vi "Mail test file V1.vi"(8 "mail file":bool, 9 "result":bool, 10 "status":string, 11 "panel id":string) -> (0 "network file save error":errorcluster, 3 "file save path":string)   [LabVIEW 2013]
uses:
  program files/Global 1.vi
panel:
  in  "mail to":string
  in  "mail from":string
  in  "mail server":string
  out "C drive root path":string
  out "network file dir path":path
  out "network dir":string
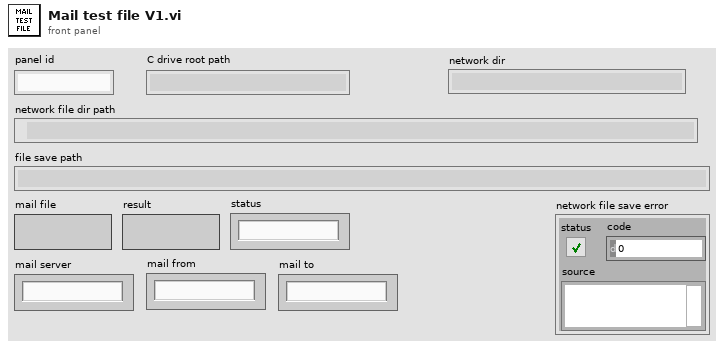
[diagram p1: front panel]
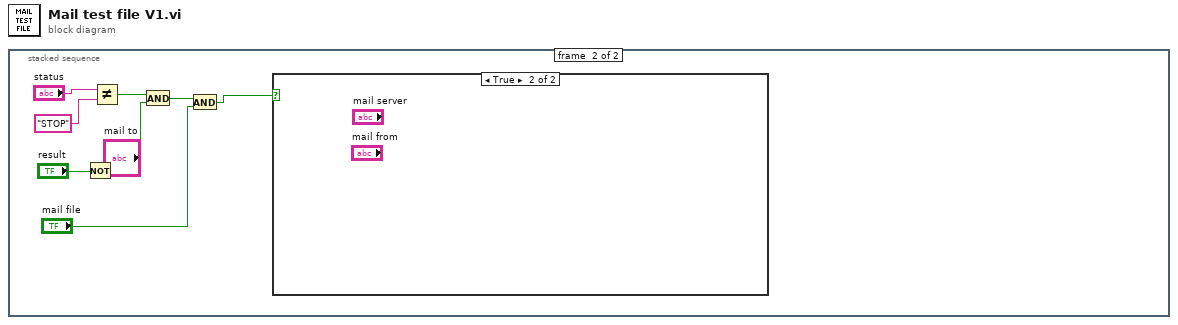
[diagram p0: block diagram]
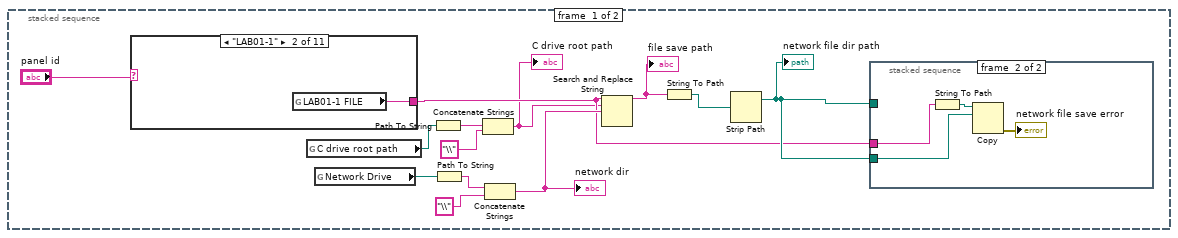
[diagram p2: hidden frame]
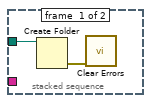
[diagram p3: hidden frame]
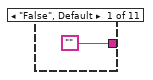
[diagram p4: hidden frame]
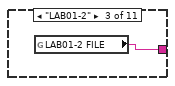
[diagram p5: hidden frame]
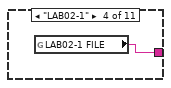
[diagram p6: hidden frame]
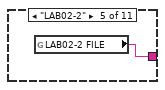
[diagram p7: hidden frame]
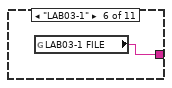
[diagram p8: hidden frame]
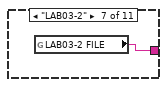
[diagram p9: hidden frame]
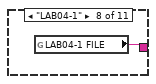
[diagram p10: hidden frame]
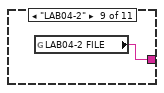
[diagram p11: hidden frame]
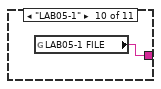
[diagram p12: hidden frame]
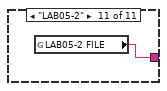
[diagram p13: hidden frame]
diagram:
  n1 = stacked-sequence {
    frame #0 {
      n2 = case shown="\"LAB01-1\"" "panel id" {
        tunnel: ["" w21 w22 w23 w24 w25 w26 w27 w28 w29 w30] -> w5
        frame "False", Default {
        }
        frame "LAB01-1" {
          n3 = global read "Global 1.vi" "LAB01-1 FILE"() -> (w21:string)
        }
        frame "LAB01-2" {
          n4 = global read "Global 1.vi" "LAB01-2 FILE"() -> (w22:string)
        }
        frame "LAB02-1" {
          n5 = global read "Global 1.vi" "LAB02-1 FILE"() -> (w23:string)
        }
        frame "LAB02-2" {
          n6 = global read "Global 1.vi" "LAB02-2 FILE"() -> (w24:string)
        }
        frame "LAB03-1" {
          n7 = global read "Global 1.vi" "LAB03-1 FILE"() -> (w25:string)
        }
        frame "LAB03-2" {
          n8 = global read "Global 1.vi" "LAB03-2 FILE"() -> (w26:string)
        }
        frame "LAB04-1" {
          n9 = global read "Global 1.vi" "LAB04-1 FILE"() -> (w27:string)
        }
        frame "LAB04-2" {
          n10 = global read "Global 1.vi" "LAB04-2 FILE"() -> (w28:string)
        }
        frame "LAB05-1" {
          n11 = global read "Global 1.vi" "LAB05-1 FILE"() -> (w29:string)
        }
        frame "LAB05-2" {
          n12 = global read "Global 1.vi" "LAB05-2 FILE"() -> (w30:string)
        }
      }
      n13 = global read "Global 1.vi" "C drive root path"() -> (w2:path)
      n14 = global read "Global 1.vi" "Network Drive"() -> (w12:path)
      n15 = Path To String(path=w2) -> (string=w3:string)
      n16 = Path To String(path=w12) -> (string=w11:string)
      n17 = Concatenate Strings(w3, "\\") -> (w1:string)
      "C drive root path" <- w1
      n18 = Concatenate Strings(w11, "\\") -> (w9:string)
      "network dir" <- w9
      n19 = Search and Replace String(input string=w5, search string=w1, replace string=w9) -> (result string=w8:string)  [unwired: 5 in, 3 out]
      "file save path" <- w8
      n20 = String To Path(string=w8) -> (path=w7:path)
      n21 = Strip Path(path=w7) -> (stripped path=w6:path)  [unwired: 1 out]
      "network file dir path" <- w6
      n22 = stacked-sequence {
        tunnel: w6 -> [w15 _]
        tunnel: w5 -> [_ w17]
        tunnel: w6 -> [_ w16]
        frame #0 {
          n23 = Create Folder(path (use dialog)=w15) -> (error out=w14:errorcluster)  [unwired: 2 in, 2 out]
          n24 = call <vilib>:"Clear Errors.vi"("error in (no error)"=w14) -> ()  [unwired: 6 in, 1 out]
        }
        frame #1 {
          n25 = String To Path(string=w17) -> (path=w18:path)
          n26 = Copy(10:w16, 11:w18) -> (0:→"network file save error":errorcluster)  [unwired: 3 in, 2 out]
        }
      }
    }
    frame #1 {
      n27 = Not(x="result") -> (.not. x?=w35:bool)
      n28 = Not Equal?(x="status", y="STOP") -> (x != y?=w34:bool)
      n29 = And(x=w34, y=w35) -> (x .and. y?=w33:bool)
      n30 = And(x=w33, y="mail file") -> (x .and. y?=w31:bool)
      n31 = case shown="True" w31 {
        frame False {
        }
        frame True {
        }
      }
    }
  }
